vi "oax_Get Channel Info (DAQmx).vi"(8 "error in (no error)":errorcluster, 9 "tachometer channel":u16(ring) items=["ch 0", "ch 1", "ch 2", "ch 3", "ch 4", "ch 5", "ch 6", "ch 7", "digital tacho"], 11 "master":T4={"DSA Device"="", "Channels"={"enable ch0"=TRUE, "enable ch1"=TRUE, "enable ch2"=FALSE, "enable ch3"=FALSE, "enable ch4"=FALSE, "enable ch5"=FALSE, "enable ch6"=FALSE, "enable ch7"=FALSE}, "Channel Names"={"ch0 string"="Tachometer", "ch1 string"="Acc1", "ch2 string"="", "ch3 string"="", "ch4 string"="", "ch5 string"="", "ch6 string"="", "ch7 string"=""}, "Coupling"={"coupling ch0"=FALSE, "coupling ch1"=FALSE, "coupling ch2"=FALSE, "coupling ch3"=FALSE, "coupling ch4"=FALSE, "coupling ch5"=FALSE, "coupling ch6"=FALSE, "coupling ch7"=FALSE}, "IEPE"={"ICP ch0"=TRUE, "ICP ch0"=FALSE, "ICP ch0"=FALSE, "ICP ch0"=FALSE, "ICP ch0"=FALSE, "ICP ch0"=FALSE, "ICP ch0"=FALSE, "ICP ch0"=FALSE}, "Ch. Sensitivity\n[mV/EU]"={"ch0 sensitivity"=1000.0, "ch1 sensitivity"=1000.0, "ch2 sensitivity"=1000.0, "ch3 sensitivity"=1000.0, "ch4 sensitivity"=1000.0, "ch5 sensitivity"=1000.0, "ch6 sensitivity"=1000.0, "ch7 sensitivity"=1000.0}, "Engineering\nUnits"={"Engineering\nUnits"=1000, "Engineering\nUnits"=100, "Engineering\nUnits"=1000, "Engineering\nUnits"=1000, "Engineering\nUnits"=1000, "Engineering\nUnits"=1000, "Engineering\nUnits"=1000, "Engineering\nUnits"=1000}, "Custom\nLabel"={"Custom Label"="", "Custom Label"="", "Custom Label"="", "Custom Label"="", "Custom Label"="", "Custom Label"="", "Custom Label"="", "Custom Label"=""}, "dB reference\n[EU]"={"dB reference [EU]"=1.0, "dB reference [EU]"=1.0, "dB reference [EU]"=1.0, "dB reference [EU]"=1.0, "dB reference [EU]"=1.0, "dB reference [EU]"=1.0, "dB reference [EU]"=1.0, "dB reference [EU]"=1.0}, "pregain\n[dB]"={"pregain [dB]"=1.0, "pregain [dB]"=1.0, "pregain [dB]"=1.0, "pregain [dB]"=1.0, "pregain [dB]"=1.0, "pregain [dB]"=1.0, "pregain [dB]"=1.0, "pregain [dB]"=1.0}, "Weighting\nFilter"={"Weighting Filter"=1, "Weighting Filter"=1, "Weighting Filter"=1, "Weighting Filter"=1, "Weighting Filter"=1, "Weighting Filter"=1, "Weighting Filter"=1, "Weighting Filter"=1}, "max value"=5.0, "min value"=5.0, "enable EAR?"=FALSE} {"min value" format="%0.2f"; "max value" format="%0.2f"; "Weighting\nFilter"."Weighting Filter" items=["Linear", "A-weighting", "B-weighting", "C-weighting", "ITU-R 468-4", "Dolby", "CCITT", "C-message"]; "Weighting\nFilter"."Weighting Filter" items=["Linear", "A-weighting", "B-weighting", "C-weighting", "ITU-R 468-4", "Dolby", "CCITT", "C-message"]; "Weighting\nFilter"."Weighting Filter" items=["Linear", "A-weighting", "B-weighting", "C-weighting", "ITU-R 468-4", "Dolby", "CCITT", "C-message"]; "Weighting\nFilter"."Weighting Filter" items=["Linear", "A-weighting", "B-weighting", "C-weighting", "ITU-R 468-4", "Dolby", "CCITT", "C-message"]; "Weighting\nFilter"."Weighting Filter" items=["Linear", "A-weighting", "B-weighting", "C-weighting", "ITU-R 468-4", "Dolby", "CCITT", "C-message"]; "Weighting\nFilter"."Weighting Filter" items=["Linear", "A-weighting", "B-weighting", "C-weighting", "ITU-R 468-4", "Dolby", "CCITT", "C-message"]; "Weighting\nFilter"."Weighting Filter" items=["Linear", "A-weighting", "B-weighting", "C-weighting", "ITU-R 468-4", "Dolby", "CCITT", "C-message"]; "Weighting\nFilter"."Weighting Filter" items=["Linear", "A-weighting", "B-weighting", "C-weighting", "ITU-R 468-4", "Dolby", "CCITT", "C-message"]; "pregain\n[dB]"."pregain [dB]" format="%.2f"; "pregain\n[dB]"."pregain [dB]" format="%.2f"; "pregain\n[dB]"."pregain [dB]" format="%.2f"; "pregain\n[dB]"."pregain [dB]" format="%.2f"; "pregain\n[dB]"."pregain [dB]" format="%.2f"; "pregain\n[dB]"."pregain [dB]" format="%.2f"; "pregain\n[dB]"."pregain [dB]" format="%.2f"; "pregain\n[dB]"."pregain [dB]" format="%.2f"; "dB reference\n[EU]"."dB reference [EU]" format="%^.1e"; "dB reference\n[EU]"."dB reference [EU]" format="%^.1e"; "dB reference\n[EU]"."dB reference [EU]" format="%^.1e"; "dB reference\n[EU]"."dB reference [EU]" format="%^.1e"; "dB reference\n[EU]"."dB reference [EU]" format="%^.1e"; "dB reference\n[EU]"."dB reference [EU]" format="%^.1e"; "dB reference\n[EU]"."dB reference [EU]" format="%^.1e"; "dB reference\n[EU]"."dB reference [EU]" format="%^.1e"; "Engineering\nUnits"."Engineering\nUnits" items=["custom..."=0, "V"=1, "A"=21, "Pa"=2, "N"=20, "g"=3, "m/s^2"=4, "m/s"=5, "m"=6, "mm/s"=12, "mm"=13, "microns/s"=14, "microns"=15, "in/s^2"=7, "in/s"=8, "in"=9, "mils/s"=10, "mils"=11, "rad/s^2"=16, "rad/s"=17, "rad"=18, "strain"=19]; "Engineering\nUnits"."Engineering\nUnits" items=["custom..."=0, "V"=1, "A"=21, "Pa"=2, "N"=20, "g"=3, "m/s^2"=4, "m/s"=5, "m"=6, "mm/s"=12, "mm"=13, "microns/s"=14, "microns"=15, "in/s^2"=7, "in/s"=8, "in"=9, "mils/s"=10, "mils"=11, "rad/s^2"=16, "rad/s"=17, "rad"=18, "strain"=19]; "Engineering\nUnits"."Engineering\nUnits" items=["custom..."=0, "V"=1, "A"=21, "Pa"=2, "N"=20, "g"=3, "m/s^2"=4, "m/s"=5, "m"=6, "mm/s"=12, "mm"=13, "microns/s"=14, "microns"=15, "in/s^2"=7, "in/s"=8, "in"=9, "mils/s"=10, "mils"=11, "rad/s^2"=16, "rad/s"=17, "rad"=18, "strain"=19]; "Engineering\nUnits"."Engineering\nUnits" items=["custom..."=0, "V"=1, "A"=21, "Pa"=2, "N"=20, "g"=3, "m/s^2"=4, "m/s"=5, "m"=6, "mm/s"=12, "mm"=13, "microns/s"=14, "microns"=15, "in/s^2"=7, "in/s"=8, "in"=9, "mils/s"=10, "mils"=11, "rad/s^2"=16, "rad/s"=17, "rad"=18, "strain"=19]; "Engineering\nUnits"."Engineering\nUnits" items=["custom..."=0, "V"=1, "A"=21, "Pa"=2, "N"=20, "g"=3, "m/s^2"=4, "m/s"=5, "m"=6, "mm/s"=12, "mm"=13, "microns/s"=14, "microns"=15, "in/s^2"=7, "in/s"=8, "in"=9, "mils/s"=10, "mils"=11, "rad/s^2"=16, "rad/s"=17, "rad"=18, "strain"=19]; "Engineering\nUnits"."Engineering\nUnits" items=["custom..."=0, "V"=1, "A"=21, "Pa"=2, "N"=20, "g"=3, "m/s^2"=4, "m/s"=5, "m"=6, "mm/s"=12, "mm"=13, "microns/s"=14, "microns"=15, "in/s^2"=7, "in/s"=8, "in"=9, "mils/s"=10, "mils"=11, "rad/s^2"=16, "rad/s"=17, "rad"=18, "strain"=19]; "Engineering\nUnits"."Engineering\nUnits" items=["custom..."=0, "V"=1, "A"=21, "Pa"=2, "N"=20, "g"=3, "m/s^2"=4, "m/s"=5, "m"=6, "mm/s"=12, "mm"=13, "microns/s"=14, "microns"=15, "in/s^2"=7, "in/s"=8, "in"=9, "mils/s"=10, "mils"=11, "rad/s^2"=16, "rad/s"=17, "rad"=18, "strain"=19]; "Engineering\nUnits"."Engineering\nUnits" items=["custom..."=0, "V"=1, "A"=21, "Pa"=2, "N"=20, "g"=3, "m/s^2"=4, "m/s"=5, "m"=6, "mm/s"=12, "mm"=13, "microns/s"=14, "microns"=15, "in/s^2"=7, "in/s"=8, "in"=9, "mils/s"=10, "mils"=11, "rad/s^2"=16, "rad/s"=17, "rad"=18, "strain"=19]; "Ch. Sensitivity\n[mV/EU]"."ch7 sensitivity" format="%.2f"; "Ch. Sensitivity\n[mV/EU]"."ch6 sensitivity" format="%.2f"; "Ch. Sensitivity\n[mV/EU]"."ch5 sensitivity" format="%.2f"; "Ch. Sensitivity\n[mV/EU]"."ch4 sensitivity" format="%.2f"; "Ch. Sensitivity\n[mV/EU]"."ch3 sensitivity" format="%.2f"; "Ch. Sensitivity\n[mV/EU]"."ch2 sensitivity" format="%.2f"; "Ch. Sensitivity\n[mV/EU]"."ch1 sensitivity" format="%.2f"; "Ch. Sensitivity\n[mV/EU]"."ch0 sensitivity" format="%.2f"}) -> (0 "error out":errorcluster, 1 "tachometer channel out":u16(ring) items=["ch 0", "ch 1", "ch 2", "ch 3", "ch 4", "ch 5", "ch 6", "ch 7", "digital tacho"], 2 "channel name":string[](array[string]), 3 "channel info":T1[](array[typedef]) {"pregain" format="%.2f"; "weighting filter" items=["Linear", "A-weighting", "B-weighting", "C-weighting", "ITU-R 468-4", "Dolby", "CCITT", "C-message", "Wb", "Wc", "Wd", "We", "Wf", "Wh", "Wj", "Wk", "Wm", "AES17 20 kHz lowpass", "AES17 40 kHz lowpass", "AES17 20 kHz highpass", "AES17 40 kHz highpass"]; "dB reference" format="%^.1e"; "engineering units" items=["custom..."=0, "V"=1, "A"=21, "C"=30, "pC"=31, "s"=32, "-"=29, "Pa"=2, "N"=20, "g"=3, "m/s^2"=4, "m/s"=5, "m"=6, "mm/s"=12, "mm"=13, "micron/s"=14, "micron"=15, "in/s^2"=7, "in/s"=8, "in"=9, "mil/s"=10, "mil"=11, "rad/s^2"=16, "rad/s"=17, "rad"=18, "deg/s^2"=26, "deg/s"=27, "deg"=28, "RPM"=22, "cycle/s^2"=23, "Hz"=24, "cycle"=25, "strain"=19]; "sensor sensitivity" format="%#_5f"}, 4 "tacho channel index":i32)   [LabVIEW 2017]
doc: "Configure and organize channel information."
uses:
  <vilib>/addons/Sound and Vibration/Order Analysis/Example Support/sub VIs/OAXML_Analog Channel Config (DAQmx).ctl
  <vilib>/addons/_NISVFA/_Shared subVIs/Controls/svc_Channel Info.ctl
  <vilib>/addons/_NISVFA/_Shared subVIs/Controls/svc_Engineering Units Text Ring.ctl
  <vilib>/addons/_NISVFA/_Shared subVIs/Controls/svc_Weighting Filter Text Ring.ctl
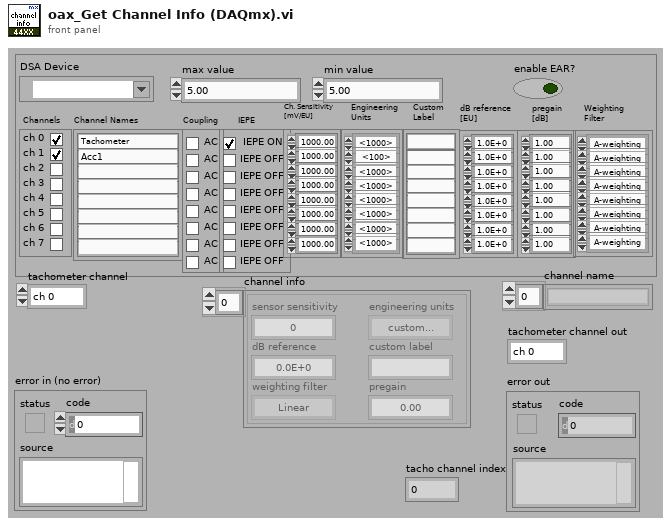
[diagram p1: front panel]
types:
  T1 = typedef "svc_Channel Info.ctl" = cluster{"sensor sensitivity":dbl, "engineering units":T2, "dB reference":dbl, "custom label":string, "weighting filter":T3, "pregain":dbl}
  T2 = typedef "svc_Engineering Units Text Ring.ctl" = u16
  T3 = typedef "svc_Weighting Filter Text Ring.ctl" = u16
  T4 = typedef "OAXML_Analog Channel Config (DAQmx).ctl" = cluster{"DSA Device":tag, "Channels":cluster{"enable ch0":bool, "enable ch1":bool, "enable ch2":bool, "enable ch3":bool, "enable ch4":bool, "enable ch5":bool, "enable ch6":bool, "enable ch7":bool}, "Channel Names":cluster{"ch0 string":string, "ch1 string":string, "ch2 string":string, "ch3 string":string, "ch4 string":string, "ch5 string":string, "ch6 string":string, "ch7 string":string}, "Coupling":cluster{"coupling ch0":bool, "coupling ch1":bool, "coupling ch2":bool, "coupling ch3":bool, "coupling ch4":bool, "coupling ch5":bool, "coupling ch6":bool, "coupling ch7":bool}, "IEPE":cluster{"ICP ch0":bool, "ICP ch0":bool, "ICP ch0":bool, "ICP ch0":bool, "ICP ch0":bool, "ICP ch0":bool, "ICP ch0":bool, "ICP ch0":bool}, "Ch. Sensitivity\n[mV/EU]":cluster{"ch0 sensitivity":dbl, "ch1 sensitivity":dbl, "ch2 sensitivity":dbl, "ch3 sensitivity":dbl, "ch4 sensitivity":dbl, "ch5 sensitivity":dbl, "ch6 sensitivity":dbl, "ch7 sensitivity":dbl}, "Engineering\nUnits":cluster{"Engineering\nUnits":u16, "Engineering\nUnits":u16, "Engineering\nUnits":u16, "Engineering\nUnits":u16, "Engineering\nUnits":u16, "Engineering\nUnits":u16, "Engineering\nUnits":u16, "Engineering\nUnits":u16}, "Custom\nLabel":cluster{"Custom Label":string, "Custom Label":string, "Custom Label":string, "Custom Label":string, "Custom Label":string, "Custom Label":string, "Custom Label":string, "Custom Label":string}, "dB reference\n[EU]":cluster{"dB reference [EU]":dbl, "dB reference [EU]":dbl, "dB reference [EU]":dbl, "dB reference [EU]":dbl, "dB reference [EU]":dbl, "dB reference [EU]":dbl, "dB reference [EU]":dbl, "dB reference [EU]":dbl}, "pregain\n[dB]":cluster{"pregain [dB]":dbl, "pregain [dB]":dbl, "pregain [dB]":dbl, "pregain [dB]":dbl, "pregain [dB]":dbl, "pregain [dB]":dbl, "pregain [dB]":dbl, "pregain [dB]":dbl}, "Weighting\nFilter":cluster{"Weighting Filter":u16, "Weighting Filter":u16, "Weighting Filter":u16, "Weighting Filter":u16, "Weighting Filter":u16, "Weighting Filter":u16, "Weighting Filter":u16, "Weighting Filter":u16}, "max value":dbl, "min value":dbl, "enable EAR?":bool}
  T5 = cluster{"ch0 sensitivity":dbl, "ch1 sensitivity":dbl, "ch2 sensitivity":dbl, "ch3 sensitivity":dbl, "ch4 sensitivity":dbl, "ch5 sensitivity":dbl, "ch6 sensitivity":dbl, "ch7 sensitivity":dbl}
  T6 = cluster{"Engineering\nUnits":u16, "Engineering\nUnits":u16, "Engineering\nUnits":u16, "Engineering\nUnits":u16, "Engineering\nUnits":u16, "Engineering\nUnits":u16, "Engineering\nUnits":u16, "Engineering\nUnits":u16}
  T7 = cluster{"dB reference [EU]":dbl, "dB reference [EU]":dbl, "dB reference [EU]":dbl, "dB reference [EU]":dbl, "dB reference [EU]":dbl, "dB reference [EU]":dbl, "dB reference [EU]":dbl, "dB reference [EU]":dbl}
  T8 = cluster{"Custom Label":string, "Custom Label":string, "Custom Label":string, "Custom Label":string, "Custom Label":string, "Custom Label":string, "Custom Label":string, "Custom Label":string}
  T9 = cluster{"Weighting Filter":u16, "Weighting Filter":u16, "Weighting Filter":u16, "Weighting Filter":u16, "Weighting Filter":u16, "Weighting Filter":u16, "Weighting Filter":u16, "Weighting Filter":u16}
  T10 = cluster{"pregain [dB]":dbl, "pregain [dB]":dbl, "pregain [dB]":dbl, "pregain [dB]":dbl, "pregain [dB]":dbl, "pregain [dB]":dbl, "pregain [dB]":dbl, "pregain [dB]":dbl}
  T11 = cluster{"ch0 string":string, "ch1 string":string, "ch2 string":string, "ch3 string":string, "ch4 string":string, "ch5 string":string, "ch6 string":string, "ch7 string":string}
  T12 = cluster{"enable ch0":bool, "enable ch1":bool, "enable ch2":bool, "enable ch3":bool, "enable ch4":bool, "enable ch5":bool, "enable ch6":bool, "enable ch7":bool}
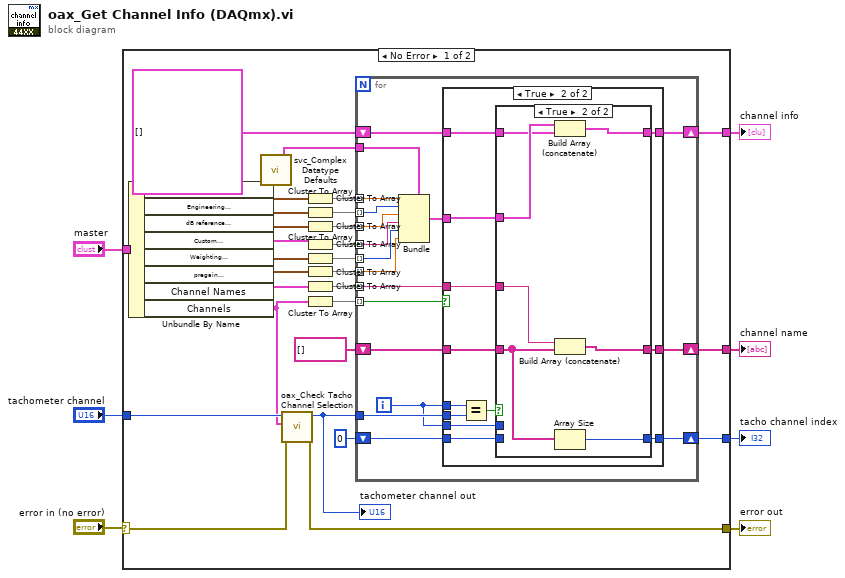
[diagram p0: block diagram]
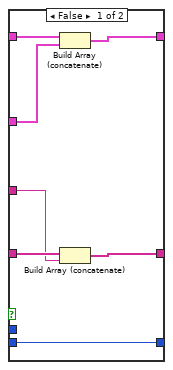
[diagram p3: hidden frame]
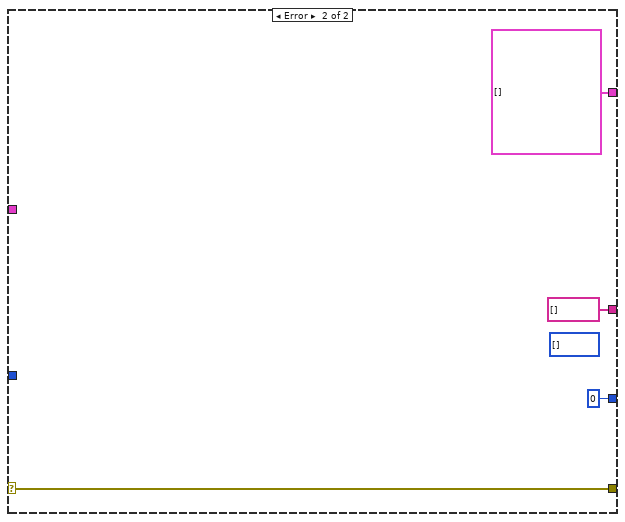
[diagram p4: hidden frame]
diagram:
  n1 = case shown="No Error" "error in (no error)" {
    selector: "error in (no error)" -> [w11 w86]
    tunnel: "master" -> [w20 _]
    tunnel: [w19 T1[] []] -> w1
    tunnel: [w17 string[] []] -> w6
    tunnel: [w10 w86] -> w4
    tunnel: "tachometer channel" -> [w12 _]
    tunnel: [w15 0] -> w2
    frame No Error {
      n2 = Unbundle By Name(w20) -> ("Ch. Sensitivity\n[mV/EU]"=w35:T5, "Engineering\nUnits"=w33:T6, "dB reference\n[EU]"=w32:T7, "Custom\nLabel"=w31:T8, "Weighting\nFilter"=w30:T9, "pregain\n[dB]"=w29:T10, "Channel Names"=w23:T11, "Channels"=w9:T12)
      n3 = call <vilib>:"svc_Complex Datatype Defaults.vi"() -> ("channel info"=w14:T1)  [unwired: 11 in, 8 out]
      n4 = call <vilib>:"oax_Check Tacho Channel Selection.vi"("error in (no error)"=w11, "Channels"=w9, "tachometer channel"=w12) -> ("error out"=w10:errorcluster, "tachometer channel out"=w8:u16)  [unwired: 7 in]
      "tachometer channel out" <- w8
      n5 = Cluster To Array(cluster=w35) -> (array=w34:dbl[])
      n6 = Cluster To Array(cluster=w33) -> (array=w28:u16[])
      n7 = Cluster To Array(cluster=w32) -> (array=w27:dbl[])
      n8 = Cluster To Array(cluster=w31) -> (array=w26:string[])
      n9 = Cluster To Array(cluster=w30) -> (array=w25:u16[])
      n10 = Cluster To Array(cluster=w29) -> (array=w24:dbl[])
      n11 = Cluster To Array(cluster=w23) -> (array=w21:string[])
      n12 = Cluster To Array(cluster=w9) -> (array=w22:bool[])
      n13 = for {
        tunnel: w34 -> [w53] mode=indexing
        tunnel: w28 -> [w52] mode=indexing
        tunnel: w27 -> [w51] mode=indexing
        tunnel: w26 -> [w50] mode=indexing
        tunnel: w25 -> [w49] mode=indexing
        tunnel: w24 -> [w48] mode=indexing
        tunnel: w22 -> [w47] mode=indexing
        shift-right: [w44] -> w19
        shift-left: T1[] [] -> [w45]
        tunnel: w21 -> [w43] mode=indexing
        shift-right: [w41] -> w17
        shift-left: string[] [] -> [w42]
        tunnel: w8 -> [w40]
        shift-right: [w38] -> w15
        shift-left: 0 -> [w37]
        tunnel: w14 -> [w36]
        i -> [w39]
        n14 = Bundle(cluster=w36, "sensor sensitivity"=w53, "engineering units"=w52, "dB reference"=w51, "custom label"=w50, "weighting filter"=w49, "pregain"=w48) -> (w46:T1)
        n15 = case shown="True" w47 {
          tunnel: w46 -> [_ w66]
          tunnel: w45 -> [w56 w68]
          tunnel: [w56 w67] -> w44
          tunnel: w43 -> [_ w63]
          tunnel: w42 -> [w55 w65]
          tunnel: [w55 w64] -> w41
          tunnel: w39 -> [_ w62]
          tunnel: w40 -> [_ w61]
          tunnel: w39 -> [_ w59]
          tunnel: [w54 w58] -> w38
          tunnel: w37 -> [w54 w57]
          frame False {
          }
          frame True {
            n16 = Equal?(x=w62, y=w61) -> (x = y?=w60:bool)
            n17 = case shown="True" w60 {
              tunnel: w68 -> [w75 w81]
              tunnel: [w74 w80] -> w67
              tunnel: w66 -> [w73 w82]
              tunnel: w65 -> [w72 w77]
              tunnel: [w71 w78] -> w64
              tunnel: w63 -> [w70 w79]
              tunnel: w59 -> [_ _]
              tunnel: [w69 w76] -> w58
              tunnel: w57 -> [w69 _]
              frame False {
                n18 = Build Array (concatenate)(w75, w73) -> (w74:T1[])
                n19 = Build Array (concatenate)(w72, w70) -> (w71:string[])
              }
              frame True {
                n20 = Build Array (concatenate)(w82, w81) -> (w80:T1[])
                n21 = Build Array (concatenate)(w79, w77) -> (w78:string[])
                n22 = Array Size(array=w77) -> (size(s)=w76:i32)
              }
            }
          }
        }
      }
    }
    frame Error {
      (unwired) u32[] []
    }
  }
  "channel name" <- w6
  "error out" <- w4
  "tacho channel index" <- w2
  "channel info" <- w1
